vi "New (1B).vi"(8 "error in (no error)":errorcluster, 10 "count (1)":u64=1, 11 "Pointer type":refnum<class "Pointer.lvclass">) -> (0 "error out":errorcluster, 3 "Pointer":refnum<class "Pointer.lvclass">)   [LabVIEW 2016, in "Memory Manager.lvlib" / "Pointer.lvclass"]
uses:
  Pointer.lvclass
  Pointer.lvclass/Pointer.ctl
  Set Address.vi
  Set Size.vi
  Set Internal.vi
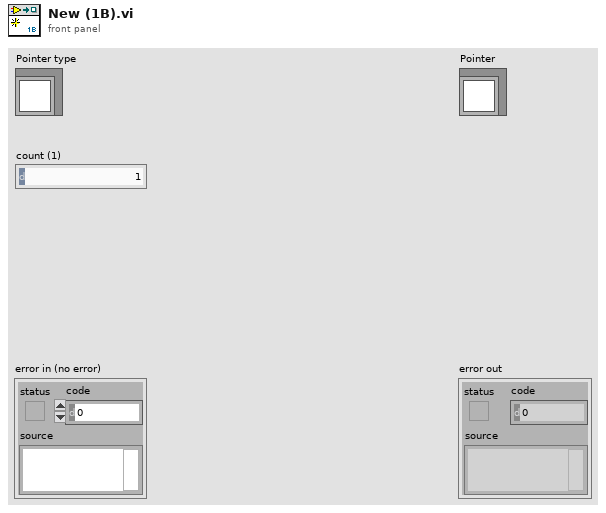
[diagram p1: front panel]
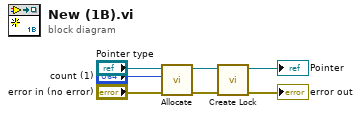
[diagram p0: block diagram]
diagram:
  n1 = call "Allocate.vi"("error in (no error)"="error in (no error)", "size"="count (1)", "Pointer in"="Pointer type") -> ("error out"=w3:errorcluster, "Pointer out"=w4:refnum<class "Pointer.lvclass">)  [unwired: 7 in]
  n2 = call-dynamic "Create Lock.vi"("error in (no error)"=w3, "Pointer in"=w4) -> ("error out"=→"error out":errorcluster, "Pointer out"=→"Pointer":refnum<class "Pointer.lvclass">)  [unwired: 8 in]
